vi "9478_Initialize.vi"(8 "error in (no error)":errorcluster, 9 "Slot Settings":T1, 11 "9478 in":refnum<class "9478.lvclass">) -> (0 "error out":errorcluster, 3 "9478 out":refnum<class "9478.lvclass">)   [LabVIEW 2011, in "Modules.lvlib" / "9478.lvclass"]
uses:
  9478.lvclass
  RSI Module/Slot Settings.ctl
  RSI Module/Module Models.ctl
  RSI Module/Channels.ctl
  RSI Module/Channel Type.ctl
  Active Limit.ctl
  9478.lvclass/9478.ctl
  RSI Module/RSI Module.lvclass
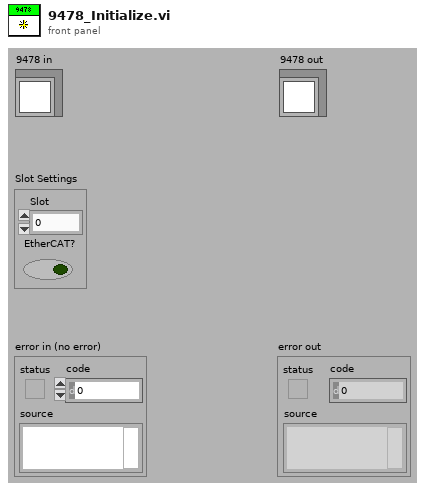
[diagram p1: front panel]
types:
  T1 = typedef "Modules.lvlib/RSI Module.lvclass/Slot Settings.ctl" = cluster{"Slot":u32, "EtherCAT?":bool}
  T2 = typedef "Modules.lvlib/RSI Module.lvclass/Module Models.ctl" = enum16{"Empty", "NI 9201", "NI 9203", "NI 9205", "NI 9206", "NI 9207", "NI 9208", "NI 9211", "NI 9213", "NI 9214", "NI 9215", "NI 9217", "NI 9219", "NI 9221", "NI 9225", "NI 9227", "NI 9229", "NI 9233", "NI 9234", "NI 9235", "NI 9236", "NI 9237", "NI 9239", "NI 9263", "NI 9264", "NI 9265", "NI 9269", "NI 9375", "NI 9401", "NI 9402", "NI 9403", "NI 9411", "NI 9421", "NI 9422", "NI 9423", "NI 9425", "NI 9426", "NI 9435", "NI 9472", "NI 9474", "NI 9475", "NI 9476", "NI 9477", "NI 9478", "NI 9481", "NI 9482", "NI 9485"}
  T3 = typedef "Modules.lvlib/RSI Module.lvclass/Channels.ctl" = cluster{"# Input Channels":i32, "# Output Channels":i32, "Channel Type":T4, "Units":string}
  T4 = typedef "Modules.lvlib/RSI Module.lvclass/Channel Type.ctl" = enum16{"Analog", "Digital"}
  T5 = typedef "Modules.lvlib/9478.lvclass/Active Limit.ctl" = u8
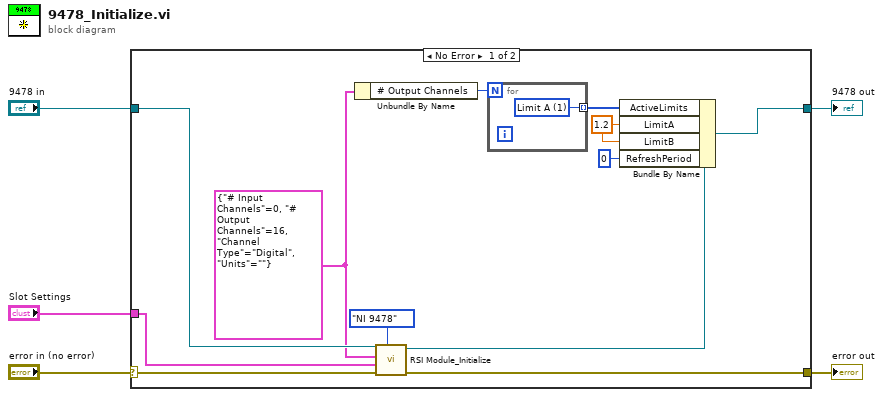
[diagram p0: block diagram]
diagram:
  n1 = case shown="No Error" "error in (no error)" {
    selector: "error in (no error)" -> [w15 w20]
    tunnel: [w14 w20] -> w4
    tunnel: [w12 w19] -> w2
    tunnel: "9478 in" -> [w17 w19]
    tunnel: "Slot Settings" -> [w16 _]
    frame No Error {
      w7 = 1.2 ("LimitA")
      w10 = T3 {"# Input Channels"=0, "# Output Channels"=16, "Channel Type"=enum."Digital", "Units"=""} ("Channels")
      n2 = Unbundle By Name(w10) -> ("# Output Channels"=w9:i32)
      n3 = call "RSI Module_Initialize.vi"("Module Model"=Module_Models."NI 9478", "error in (no error)"=w15, "Slot Settings"=w16, "Channels"=w10, "RSI Module in"=w17) -> ("error out"=w14:errorcluster, "RSI Module out"=w13:refnum<class "9478.lvclass">)  [unwired: 5 in]
      n4 = for {
        N: w9 -> [_]
        tunnel: [w18] -> w8 mode=indexing
        w18 = T5 1 items=["Limit A"=1, "Limit B"=2, "No Limit"=3] ("Active Limit")
      }
      n5 = Bundle By Name(cluster=w13, "ActiveLimits"=w8, "LimitA"=w7, "LimitB"=w7, "RefreshPeriod"=u8 0) -> (w12:refnum<class "9478.lvclass">)
    }
    frame Error {
    }
  }
  "error out" <- w4
  "9478 out" <- w2
